vi "SVPO Order Metrics for Periodic Inspection.vi"   [LabVIEW 2017, in "SoundVib_OrderTracking.lvlib"]
doc: "Computes the metrics of designated orders in an even-angle signal, such as magnitudes, phases, speed, DC gap, RMS level, and max-min level. This VI calculates metrics values from the latest integration cycles of the even-angle signal. Use this VI on embedded targets that have limited computational resources. Wire data to the <B>even-angle signal</B> input to determine the polymorphic instance to use or manually select the instance."
uses:
  <vilib>/addons/Sound and Vibration/Order Analysis/Resample Order Tracking/SoundVib_OrderTracking.lvlib
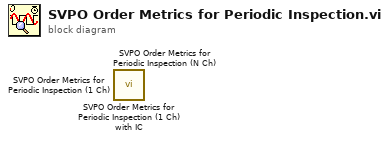
[diagram p0: block diagram]
diagram:
  n1 = call <vilib>:"SVPO Order Metrics for Periodic Inspection (1 Ch) with IC.vi"() -> ()  [unwired: 9 in, 7 out]
  n2 = call <vilib>:"SVPO Order Metrics for Periodic Inspection (N Ch).vi"() -> ()  [unwired: 10 in, 6 out]
  n3 = call <vilib>:"SVPO Order Metrics for Periodic Inspection (1 Ch).vi"() -> ()  [unwired: 10 in, 6 out]
